vi "Compute 3D Positions Relative to the Camera.vi"(4 "Camera Angle on the robot (deg)":dbl, 6 "Camera Height on robot (in)":dbl, 7 "Distance to target (in)":dbl=36.0, 10 "Thata Y":dbl, 11 "Thata Z":dbl) -> (1 "Z Corrected":dbl, 2 "Y Corrected":dbl, 3 "X (in)":dbl)   [LabVIEW 2023]
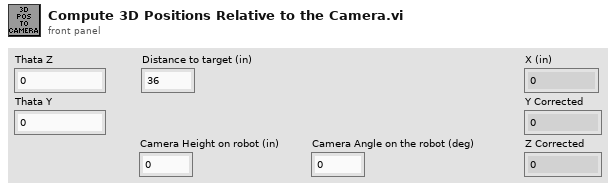
[diagram p1: front panel]
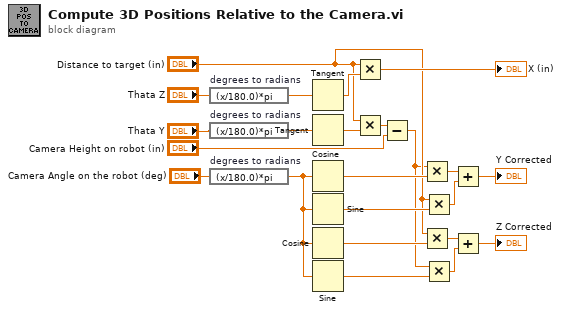
[diagram p0: block diagram]
diagram:
  n1 = expression code="(x/180.0)*pi" "degrees to radians"("Thata Z") -> (w20:dbl)
  n2 = expression code="(x/180.0)*pi" "degrees to radians"("Thata Y") -> (w19:dbl)
  n3 = expression code="(x/180.0)*pi" "degrees to radians"("Camera Angle on the robot (deg)") -> (w3:dbl)
  n4 = Tangent(1:w20) -> (0:w23:dbl)
  n5 = Tangent(1:w19) -> (0:w17:dbl)
  n6 = Cosine(x=w3) -> (cos(x)=w14:dbl)
  n7 = Sine(x=w3) -> (sin(x)=w12:dbl)
  n8 = Cosine(x=w3) -> (cos(x)=w4:dbl)
  n9 = Sine(x=w3) -> (sin(x)=w6:dbl)
  n10 = Multiply(x="Distance to target (in)", y=w23) -> (x*y=→"X (in)":dbl)
  n11 = Multiply(x="Distance to target (in)", y=w17) -> (x*y=w18:dbl)
  n12 = Subtract(x=w18, y="Camera Height on robot (in)") -> (x-y=w1:dbl)
  n13 = Multiply(x=w1, y=w14) -> (x*y=w13:dbl)
  n14 = Multiply(x="Distance to target (in)", y=w4) -> (x*y=w5:dbl)
  n15 = Multiply(x="Distance to target (in)", y=w12) -> (x*y=w11:dbl)
  n16 = Multiply(x=w1, y=w6) -> (x*y=w7:dbl)
  n17 = Add(x=w13, y=w11) -> (x+y=→"Y Corrected":dbl)
  n18 = Add(x=w5, y=w7) -> (x+y=→"Z Corrected":dbl)
